vi "USB2XXX_UART_WriteReadTest 20210727(1).vi"() -> ()   [LabVIEW 2010]
panel:
  out "pDevNum":i32[](array[numeric])
  out "pReadData":u8[](array[numeric]) format="%.0x"
  in  "pConfig":T1={"BaudRate"=115200, "WordLength"=0, "StopBits"=1, "Parity"=0, "TEPolarity"=0}
  out "Readed Data Num":i32=4
  out "Read Data(Hex)":string=" 00 00 00 E0 00 00 00 E0"
  in  "Write Data(Hex)":string="00 0A 01 42 53 4C 00 56"
  in  "Channel Index":u8(ring) items=["UART0", "UART1"]
  in  "Device Index":i32(ring) items=["0", "1", "2", "3", "4", "5"]
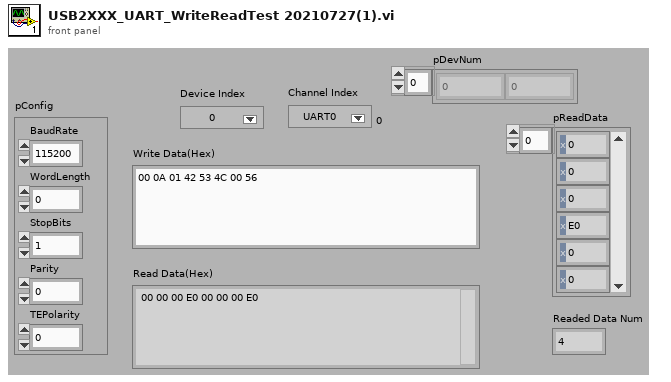
[diagram p1: front panel]
types:
  T1 = cluster{"BaudRate":u32, "WordLength":u8, "StopBits":u8, "Parity":u8, "TEPolarity":u8}
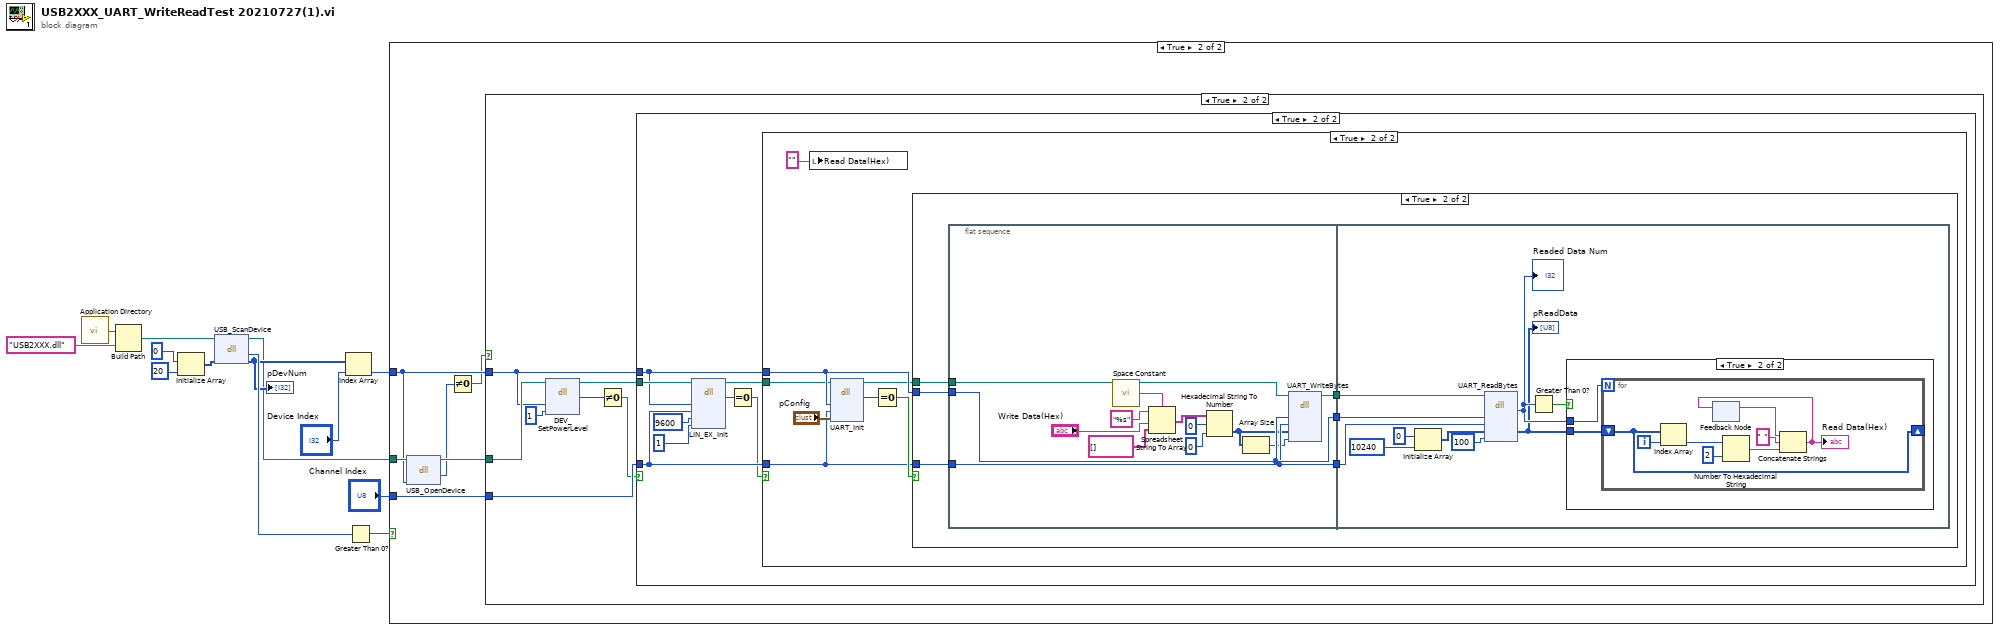
[diagram p0: block diagram]
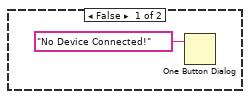
[diagram p2: hidden frame]
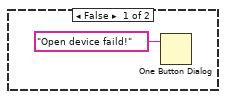
[diagram p5: hidden frame]
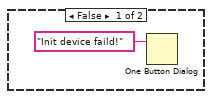
[diagram p6: hidden frame]
diagram:
  n1 = call <vilib>:"Application Directory.vi"() -> ("Application Directory"=w2:path)
  n2 = Build Path(base path=w2, name or relative path="USB2XXX.dll") -> (appended path=w1:path)
  n3 = Initialize Array(0, 20 ("dimension size")) -> (w11:i32[])
  n4 = dll-call lib="D:/yingchao li/TOOMOSS/USB2XXX_Example/sdk/api/Labview/USB2XXX.dll" fn="USB_ScanDevice"(path in=w1, "pDevNum"=w11) -> (path out=w6:path, "return type"=w10:i32, "pDevNum"=w9:i32[])  [unwired: 2 in, 1 out]
  "pDevNum" <- w9
  n5 = Index Array(array=w9, index="Device Index") -> (element=w5:i32)
  n6 = Greater Than 0?(x=w10) -> (x > 0?=w7:bool)
  n7 = case shown="True" w7 {
    tunnel: w6 -> [_ w20]
    tunnel: w5 -> [_ w18]
    tunnel: "Channel Index" -> [_ w17]
    frame False {
      n8 = One Button Dialog(message="No Device Connected!") -> ()  [unwired: 1 in, 1 out]
    }
    frame True {
      n9 = dll-call lib="D:/yingchao li/TOOMOSS/USB2XXX.dll" fn="USB_OpenDevice"(path in=w20, "DevIndex"=w18) -> (path out=w19:path, "return type"=w15:u8)  [unwired: 3 in, 1 out]
      n10 = Not Equal To 0?(x=w15) -> (x != 0?=w16:bool)
      n11 = case shown="True" w16 {
        tunnel: w19 -> [_ w26]
        tunnel: w18 -> [_ w22]
        tunnel: w17 -> [_ w27]
        frame False {
        }
        frame True {
          n12 = dll-call lib="E:/USB2XXX_Example/sdk/api/Labview/USB2XXX.*" fn="DEV_SetPowerLevel"(path in=w26, "DevHandle"=w22, "PowerLevel"=i8 1) -> (path out=w25:path, "return type"=w24:u8)  [unwired: 4 in, 1 out]
          n13 = Not Equal To 0?(x=w24) -> (x != 0?=w23:bool)
          n14 = case shown="True" w23 {
            tunnel: w25 -> [_ w35]
            tunnel: w22 -> [_ w33]
            tunnel: w27 -> [_ w32]
            frame False {
            }
            frame True {
              n15 = dll-call lib="E:/OtherWork/STM32/USB2XXX_Example/examples/Labview/PublicFiles/USB2XXX.dll" fn="LIN_EX_Init"(path in=w35, "DevHandle"=w33, "LINIndex"=w32, "BaudRate"=u32 9600, "MasterMode"=u8 1) -> (path out=w34:path, "return type"=w28:i32)  [unwired: 6 in, 1 out]
              n16 = Equal To 0?(x=w28) -> (x = 0?=w29:bool)
              n17 = case shown="True" w29 {
                tunnel: w34 -> [_ w40]
                tunnel: w33 -> [_ w42]
                tunnel: w32 -> [_ w41]
                frame False {
                  n18 = One Button Dialog(message="Open device faild!") -> ()  [unwired: 1 in, 1 out]
                }
                frame True {
                  n19 = local write "Read Data(Hex)"("" ("Read Data(Hex)")) -> ()
                  n20 = dll-call lib="E:/OtherWork/STM32/USB2XXX_Example/sdk/api/Labview/USB2XXX.*" fn="UART_Init"(path in=w40, "DevHandle"=w42, "Channel"=w41, "pConfig"="pConfig") -> (path out=w39:path, "return type"=w38:i32)  [unwired: 5 in, 1 out]
                  n21 = Equal To 0?(x=w38) -> (x = 0?=w44:bool)
                  n22 = case shown="True" w44 {
                    tunnel: w39 -> [_ w51]
                    tunnel: w42 -> [_ w50]
                    tunnel: w41 -> [_ w49]
                    frame False {
                      n23 = One Button Dialog(message="Init device faild!") -> ()  [unwired: 1 in, 1 out]
                    }
                    frame True {
                      n24 = flat-sequence {
                        tunnel: w51 -> [w57]
                        tunnel: w50 -> [w56]
                        tunnel: w49 -> [w55]
                        tunnel: [w52] -> w48
                        tunnel: [w56] -> w47
                        tunnel: [w55] -> w46
                        tunnel: w46 -> [w69]
                        tunnel: w47 -> [w70]
                        tunnel: w48 -> [w71]
                        frame #0 {
                          n25 = call <vilib>:"Space Constant.vi"() -> ("String"=w60:string)
                          n26 = Spreadsheet String To Array(delimiter (Tab)=w60, format string="%s", spreadsheet string="Write Data(Hex)", array type (2D Dbl)=string[] []) -> (array=w63:string[])
                          n27 = Hexadecimal String To Number(string=w63, offset=0, default (0uL)=u8 0 ("default (0 U32)")) -> (number=w54:u8[])  [unwired: 1 out]
                          n28 = Array Size(array=w54) -> (size(s)=w53:i32)
                          n29 = dll-call lib="E:/OtherWork/STM32/USB2XXX_Example/sdk/api/Labview/USB2XXX.*" fn="UART_WriteBytes"(path in=w57, "DevHandle"=w56, "Channel"=w55, "pWriteData"=w54, "DataSize"=w53) -> (path out=w52:path)  [unwired: 7 in, 1 out]
                        }
                        frame #1 {
                          n30 = Initialize Array(u8 0 ("element"), 10240 ("dimension size")) -> (w68:u8[])
                          n31 = dll-call lib="E:/OtherWork/STM32/USB2XXX_Example/sdk/api/Labview/USB2XXX.*" fn="UART_ReadBytes"(path in=w71, "DevHandle"=w70, "Channel"=w69, "pReadData"=w68, "TimeOutMs"=100) -> ("return type"=w66:i32, "pReadData"=w65:u8[])  [unwired: 5 in, 2 out]
                          "Readed Data Num" <- w66
                          "pReadData" <- w65
                          n32 = Greater Than 0?(x=w66) -> (x > 0?=w74:bool)
                          n33 = case shown="True" w74 {
                            tunnel: w66 -> [_ w76]
                            tunnel: w65 -> [_ w75]
                            frame False {
                            }
                            frame True {
                              n34 = for {
                                N: w76 -> [_]
                                shift-right: [w77] -> _
                                shift-left: w75 -> [w77]
                                i -> [w84]
                                n35 = Index Array(array=w77, index=w84) -> (element=w83:u8)
                                n36 = feedback #1() -> (w81:string)  [unwired: 1 in]
                                n37 = Number To Hexadecimal String(1:i16 2 ("width (-)"), 2:w83) -> (0:w79:string)
                                n38 = Concatenate Strings(w81, " " ("string"), w79) -> (w78:string)
                                "Read Data(Hex)" <- w78
                                n39 = feedback-in #1(w78) -> ()
                              }
                            }
                          }
                        }
                      }
                    }
                  }
                }
              }
            }
          }
        }
      }
    }
  }
